vi "Rename Event.vi"(8 "error in (no error)":errorcluster, 9 "eventIndex":i32, 10 "Name":string, 11 "Tosca in":refnum<class "Parameters.lvclass">) -> (0 "error out":errorcluster, 2 "Old Name":string, 3 "Tosca out":refnum<class "Parameters.lvclass">)   [LabVIEW 2015, in "Parameters.lvclass"]
uses:
  Parameters.lvclass
  Parameters.lvclass/Parameters.ctl
  State/State.lvclass
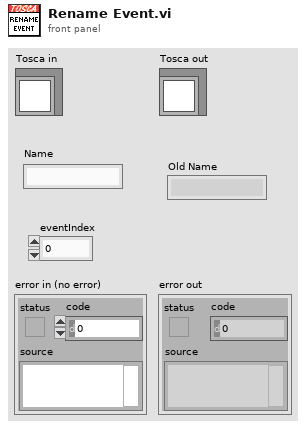
[diagram p1: front panel]
types:
  T1 = typedef "Tosca-Input Event.ctl" = cluster{"Name":string, "Criteria":T2[], "Operators":enum16{"AND", "OR"}[], "Accumulator":T4}
  T2 = typedef "Tosca-Input Criterion.ctl" = cluster{"DigInput":i32, "State":T3, "Time (ms)":i32, "Name":string}
  T3 = typedef "Logic State.ctl" = enum16{"Low", "High", "Rising", "Falling"}
  T4 = typedef "Tosca-Accumulator.ctl" = cluster{"active":bool, "N":i32, "T":dbl, "Imax":dbl, "latency":dbl}
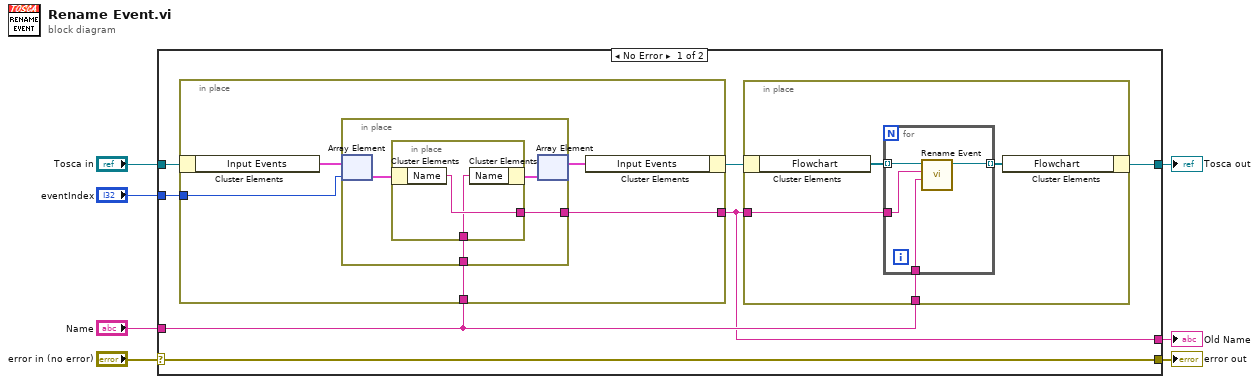
[diagram p0: block diagram]
diagram:
  n1 = case shown="No Error" "error in (no error)" {
    selector: "error in (no error)" -> [w14 w35]
    tunnel: [w14 w35] -> w6
    tunnel: [w10 w34] -> w4
    tunnel: "Tosca in" -> [w13 w34]
    tunnel: "eventIndex" -> [w12 _]
    tunnel: "Name" -> [w9 _]
    tunnel: [w8 _] -> w1
    frame No Error {
      n2 = in-place {
        in-place-border: w12 -> [w26]
        in-place-border: [w25] -> w8
        in-place-border: w9 -> [w23]
        n3 = in-place-cluster #1(w13) -> ("Input Events"=w27:T1[])
        n4 = in-place {
          in-place-border: [w30] -> w25
          in-place-border: w23 -> [w28]
          n5 = in-place-array #2(w27, w26) -> (w31:T1)
          n6 = in-place {
            in-place-border: [w33] -> w30
            in-place-border: w28 -> [w32]
            n7 = in-place-cluster #3(w31) -> ("Name"=w33:string)
            n8 = in-place-cluster #3("Name"=w32) -> (w29:T1)
          }
          n9 = in-place-array #2(w29) -> (w24:T1[])  [unwired: 1 out]
        }
        n10 = in-place-cluster #1("Input Events"=w24) -> (w11:refnum<class "Parameters.lvclass">)
      }
      n11 = in-place {
        in-place-border: w8 -> [w16]
        in-place-border: w9 -> [w15]
        n12 = in-place-cluster #4(w11) -> ("Flowchart"=w18:refnum<class "State.lvclass">[])
        n13 = for {
          tunnel: w18 -> [w22] mode=indexing
          tunnel: [w21] -> w17 mode=indexing
          tunnel: w16 -> [w20]
          tunnel: w15 -> [w19]
          n14 = call "Rename Event.vi"("New Name"=w19, "Old Name"=w20, "State in"=w22) -> ("State out"=w21:refnum<class "State.lvclass">)  [unwired: 7 in, 1 out]
        }
        n15 = in-place-cluster #4("Flowchart"=w17) -> (w10:refnum<class "Parameters.lvclass">)
      }
    }
    frame Error {
    }
  }
  "error out" <- w6
  "Tosca out" <- w4
  "Old Name" <- w1
